vi "Init.vi"(8 "error in (no error)":errorcluster, 11 "reference in":refnum<class "MES_Local.lvclass">) -> (0 "error out":errorcluster, 3 "reference out":refnum<class "MES_Local.lvclass">)   [LabVIEW 2022 SP3, in "MES_Local.lvlib" / "MES_Local.lvclass"]
uses:
  MES_Local.lvclass
  Components/Login_Base.lvlibp/Login_Base.lvclass
  Components/MES_Base.lvlibp/MES_Base.lvclass
  Components/ViPER.lvlibp/ViPER.lvclass
  C:/Projects/Medulla/ViPER/Examples/Flux_Capacitor_Tester/Components/ViPER.lvlibp/ViPER.lvclass
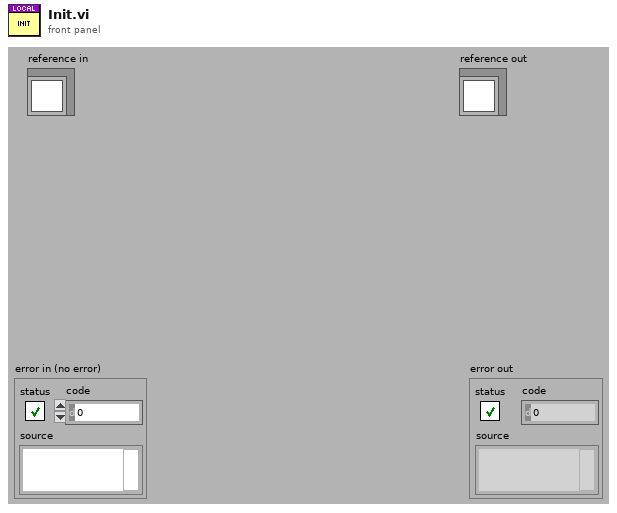
[diagram p1: front panel]
types:
  T1 = typedef "MES_Local.lvlib/MES_Local.lvclass/ObjectAttributes.ctl" = cluster{"Config":T2, "Logged_In?":bool, "AttributeNames":string[], "AttributeWritten":bool[], "ComponentNames":string[], "TestIndex":i32, "TestTag":string[], "Time Stamp":timestamp, "Employee":string, "Resource_Key":string, "Local Spec":path, "Login":refnum<class "Login_Base.lvclass">, "ReportPath":path, "Spec":T3, "StartTime":timestamp, "Role":string}
  T2 = typedef "MES_Local.lvlib/MES_Local.lvclass/Config.ctl" = cluster{"Results_Path":path}
  T3 = typedef "MES_Base.lvlibp/MES_Base.lvclass/Spec.ctl" = cluster{"Header":cluster{"Doctype":string, "Checksum":string, "DriverKey":string, "SpecId":string, "TransactionId":string, "AccountId":string, "SpecName":string, "WorkflowStep":string, "SerialNumber":string, "BatchNumber":string, "Status":enum16{"Pending", "Pass", "Fail"}, "Comment":string, "FirstFail":string, "Employee":string, "LocalMachine":string, "ResourceKey":string, "Date":string, "Time":string, "Duration":string, "DUT Position":i32}, "Components":cluster{"SerialNumber":string, "PartNumber":string, "Revision":string, "BatchNumber":string, "Name":string, "Description":string, "Attached":bool}[], "Attributes":cluster{"Name":string, "Description":string, "DataType":enum16{"NA", "String", "Boolean", "Int", "Dbl"}, "Value":variant, "DisplayFormat":string, "ReadOnly":bool, "Required":bool}[], "Tests":cluster{"Code":string, "Name":string, "Description":string, "Group":string, "IsGroup":bool, "Tag":string, "Method":string, "Parrameter":string, "DataType":enum16{"NA", "String", "Boolean", "Int", "Dbl"}, "Value":variant, "Status":enum16{"Pending", "Pass", "Fail"}, "LimitLo":variant, "LimitHi":variant, "StringMatch":string, "BooleanMatch":bool, "DisplayFormat":string, "Units":string, "TestTime":dbl}[]}
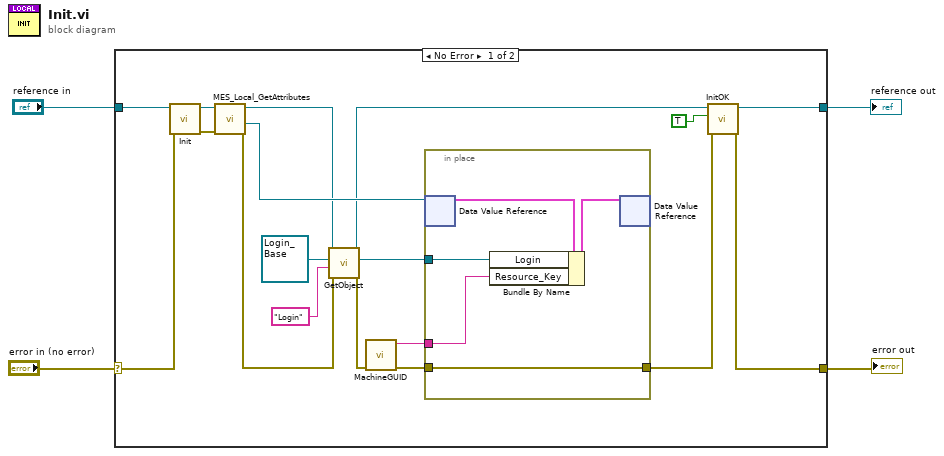
[diagram p0: block diagram]
diagram:
  n1 = case shown="No Error" "error in (no error)" {
    selector: "error in (no error)" -> [w21 w29]
    tunnel: [w14 w29] -> w3
    tunnel: [w17 w28] -> w1
    tunnel: "reference in" -> [w22 w28]
    frame No Error {
      n2 = call-parent "Init.vi"("error in (no error)"=w21, "reference in"=w22) -> ("error out"=w19:errorcluster, "reference out"=w20:refnum<class "MES_Local.lvclass">)  [unwired: 8 in]
      n3 = call "MES_Local_GetAttributes.vi"("error in (no error)"=w19, "reference in"=w20) -> ("error out"=w9:errorcluster, "DataRef"=w18:refnum<data-value>, "reference out"=w11:refnum<class "MES_Local.lvclass">)  [unwired: 6 in, 1 out]
      n4 = call "GetObject.vi"("error in (no error)"=w9, "Object Name"="Login", "Class type"=refnum<class "Login_Base.lvclass"> refnum ("Login_Base.lvlibp:reference"), "reference in"=w11) -> ("error out"=w5:errorcluster, "Object out"=w6:refnum<class "Login_Base.lvclass">, "reference out"=w10:refnum<class "MES_Local.lvclass">)  [unwired: 5 in]
      n5 = call "MachineGUID.vi"("error in (no error)"=w5) -> ("error out"=w12:errorcluster, "Machine GUID"=w13:string)  [unwired: 9 in]
      n6 = in-place {
        in-place-border: w12 -> [w27]
        in-place-border: [w27] -> w15
        in-place-border: w13 -> [w24]
        in-place-border: w6 -> [w23]
        n7 = in-place-dvr #1(w18) -> (w26:T1)  [unwired: 1 out]
        n8 = Bundle By Name(cluster=w26, "Login"=w23, "Resource_Key"=w24) -> (w25:T1)
        n9 = in-place-dvr #1(w25) -> ()  [unwired: 2 out]
      }
      n10 = call "InitOK.vi"("error in (no error)"=w15, "Init OK?"=TRUE, "reference in"=w10) -> ("error out"=w14:errorcluster, "reference out"=w17:refnum<class "MES_Local.lvclass">)  [unwired: 7 in]
    }
    frame Error {
    }
  }
  "error out" <- w3
  "reference out" <- w1
